vi "settings.vi"(6 "Param":string) -> (0 "error out":errorcluster, 2 "Rezult":string)   [LabVIEW 2010]
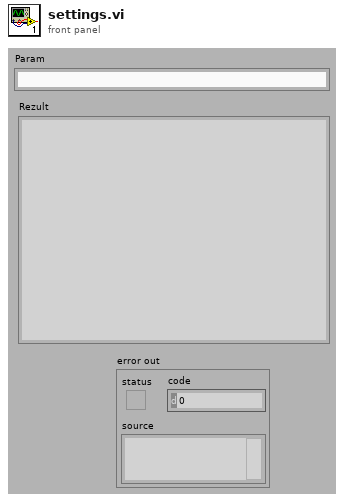
[diagram p1: front panel]
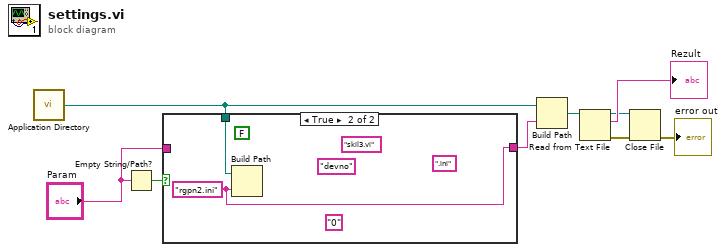
[diagram p0: block diagram]
diagram:
  n1 = call <vilib>:"Application Directory.vi"() -> ("Application Directory"=w1:path)
  n2 = Empty String/Path?(string/path="Param") -> (empty?=w4:bool)
  n3 = case shown="True" w4 {
    tunnel: "Param" -> [w10 _]
    tunnel: [w10 w11] -> w2
    tunnel: w1 -> [_ w12]
    frame False {
    }
    frame True {
      (unwired) ".ini" ("string")
      (unwired) "0"
      (unwired) "devno" ("key")
      (unwired) "skil3.vi" ("section")
      (unwired) FALSE ("create file if necessary (T)")
      w11 = "rgpn2.ini" ("name or relative path")
      n4 = Build Path(base path=w12, name or relative path=w11) -> ()  [unwired: 1 out]
    }
  }
  n5 = Build Path(base path=w1, name or relative path=w2) -> (appended path=w5:path)
  n6 = Read from Text File(file (use dialog)=w5) -> (refnum out=w6:refnum<file>, text=→"Rezult":string, error out=w8:errorcluster)  [unwired: 3 in, 1 out]
  n7 = Close File(refnum=w6, error in=w8) -> (error out=→"error out":errorcluster)  [unwired: 1 out]
